vi "Zmienne globalne.vi"() -> ()   [LabVIEW 2014]
panel:
  in  "Format_to_xsl":string="%#.6g"
  in  "opis wprost":string="Srednia("
  in  "opis modul":string="Wyprostowana("
  in  "opis kwadrat":string="Skuteczna("
  in  "Wykresy Edit":i32=1290
  in  "kolor linii":u32=26112
  in  "przezroczysty":u32=16777216
  in  "Szybka Bufor":i32=32000
  in  "Wolna Bufor":i32=32000
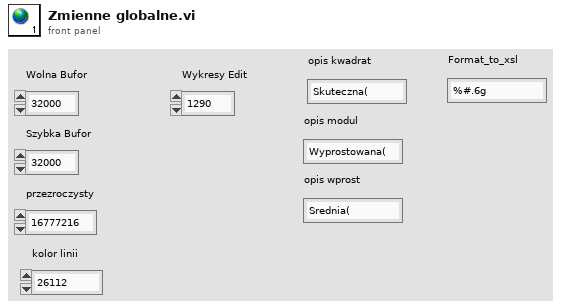
[diagram p1: front panel]
diagram:
